vi "LVIS_WriteErrorLog.vi"(7 "Success?":bool, 8 "Error In":errorcluster, 9 "Send CRC":string, 10 "DC Recieved":string, 11 "DC Sent":string) -> (0 "Error out":errorcluster)   [LabVIEW 2015]
doc: "Writes an error entry into the Data Commander error log."
uses:
  Globals/LVIS_IsGlobal.vi
  Globals/LVIS_DcGlobals.vi
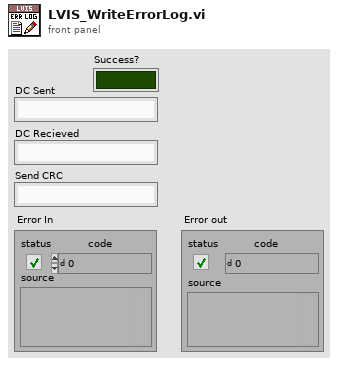
[diagram p1: front panel]
types:
  T1 = enum16{"open", "replace", "create", "open or create", "replace or create", "replace or create with confirmation"}
  T2 = cluster{"DCIP":string, "BackupFile":string, "ErrorLog":string, "FilePosition":string}
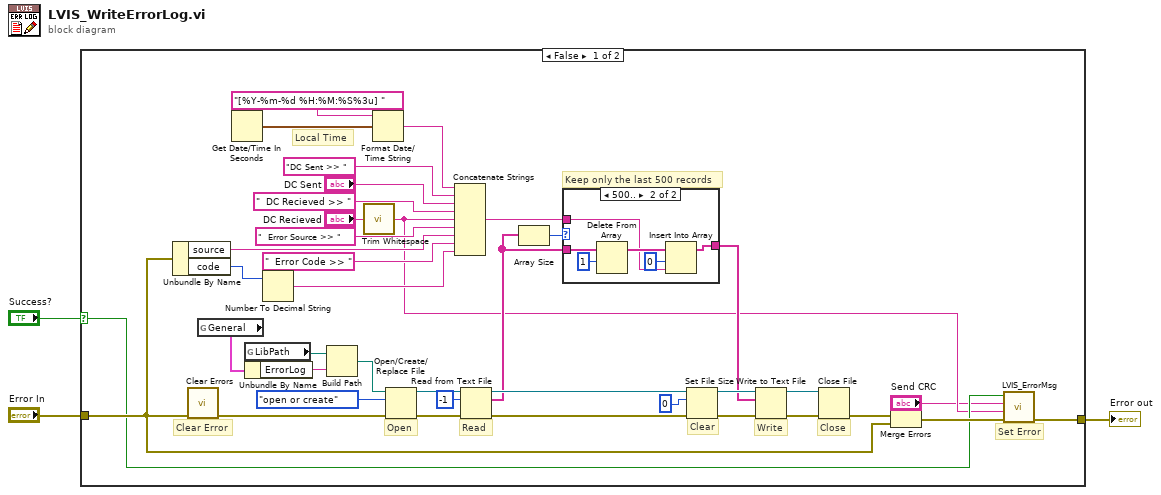
[diagram p0: block diagram]
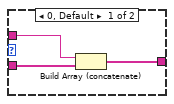
[diagram p2: hidden frame]
diagram:
  n1 = case shown="False" "Success?" {
    selector: "Success?" -> [w7 _]
    tunnel: "Error In" -> [w17 w52]
    tunnel: [w8 w52] -> w2
    frame False {
      # "Set Error"
      # "Local Time"
      # "Keep only the last 500 records"
      # "Close"
      # "Write"
      # "Clear"
      # "Read"
      # "Open"
      # "Clear Error"
      n2 = Unbundle By Name(w17) -> ("source"=w16:string, "code"=w15:i32)
      n3 = call <vilib>:"Clear Errors.vi"("error in (no error)"=w17) -> ("error out"=w42:errorcluster)  [unwired: 5 in, 1 out]
      n4 = global read "LVIS_DcGlobals.vi" "General"() -> (w12:T2)
      n5 = Get Date/Time In Seconds() -> (seconds since 1Jan1904=w37:timestamp)
      n6 = global read "LVIS_IsGlobal.vi" "LibPath"() -> (w11:path)
      n7 = Unbundle By Name(w12) -> ("ErrorLog"=w13:string)
      n8 = Number To Decimal String(number=w15) -> (decimal integer string=w14:string)  [unwired: 1 in]
      n9 = Build Path(base path=w11, name or relative path=w13) -> (appended path=w10:path)
      n10 = call <vilib>:"Trim Whitespace.vi"("string"="DC Recieved") -> ("trimmed string"=w5:string)  [unwired: 1 in]
      n11 = Format Date/Time String(time format string (%c)="[%Y-%m-%d %H:%M:%S%3u] ", seconds (now)=w37) -> (date/time string=w38:string)  [unwired: 1 in]
      n12 = Open/Create/Replace File(file path (use dialog)=w10, error in=w42, operation (0:open)=T1."open or create") -> (refnum out=w29:refnum<file>, error out=w28:errorcluster)  [unwired: 3 in, 1 out]
      n13 = Concatenate Strings(w38, "DC Sent >> ", "DC Sent", "  DC Recieved >> ", w5, "  Error Source >> ", w16, "  Error Code >> ", w14) -> (w31:string)
      n14 = Read from Text File(file (use dialog)=w29, count=-1, error in=w28) -> (refnum out=w39:refnum<file>, text=w35:string[], error out=w24:errorcluster)  [unwired: 1 in, 1 out]
      n15 = Array Size(array=w35) -> (size(s)=w27:i32)
      n16 = case shown="500.." w27 {
        tunnel: w35 -> [w45 w51]
        tunnel: w31 -> [w44 w48]
        tunnel: [w43 w47] -> w21
        frame 0, Default {
          n17 = Build Array (concatenate)(w44, w45) -> (w43:string[])
        }
        frame 500.. {
          n18 = Delete From Array(array=w51, length=1) -> (array with subset deleted=w49:string[])  [unwired: 1 in, 1 out]
          n19 = Insert Into Array(array=w49, index=0, new element=w48) -> (w47:string[])
        }
      }
      n20 = Set File Size(4:w24, 6:i64 0 ("offset (in bytes) (0)"), 7:w39) -> (0:w23:errorcluster, 3:w22:refnum<file>)
      n21 = Write to Text File(file (use dialog)=w22, text=w21, error in=w23) -> (refnum out=w25:refnum<file>, error out=w26:errorcluster)  [unwired: 1 in, 1 out]
      n22 = Close File(refnum=w25, error in=w26) -> (error out=w41:errorcluster)  [unwired: 1 out]
      n23 = Merge Errors(w41, w17) -> (w9:errorcluster)
      n24 = call "LVIS_ErrorMsg.vi"("Error In"=w9, "Response"=w5, "Send CRC"="Send CRC", "Success?"=w7) -> ("Error out"=w8:errorcluster)  [unwired: 7 in]
    }
    frame True {
    }
  }
  "Error out" <- w2
